vi "Transplantation_of_Description_field.vi"() -> ()   [LabVIEW 2018]
panel:
  out "error out":errorcluster
  in  "TDMS acceptor path":path
  in  "TDMS donor path":path
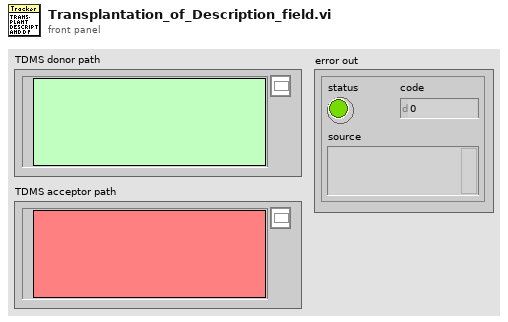
[diagram p1: front panel]
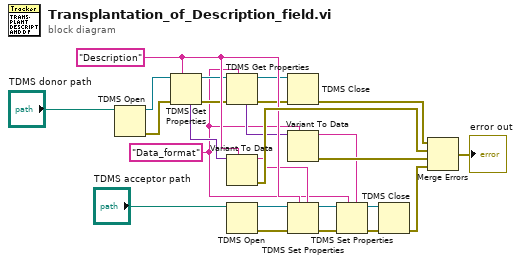
[diagram p0: block diagram]
diagram:
  w6 = "Data_format" ("property name")
  w16 = "Description" ("property name")
  n1 = TDMS Open(11:"TDMS donor path") -> (0:w24:errorcluster, 3:w25:refnum<k34>)  [unwired: 6 in]
  n2 = TDMS Get Properties(7:w16, 8:w24, 11:w25) -> (0:w11:errorcluster, 3:w13:refnum<k34>, 4:w22:variant)  [unwired: 3 in, 3 out]
  n3 = TDMS Get Properties(7:w6, 8:w11, 11:w13) -> (0:w10:errorcluster, 3:w12:refnum<k34>, 4:w9:variant)  [unwired: 3 in, 3 out]
  n4 = Variant To Data(type=w16, Variant=w22) -> (data=w15:string, error out=w20:errorcluster)  [unwired: 1 in]
  n5 = TDMS Open(11:"TDMS acceptor path") -> (0:w17:errorcluster, 3:w18:refnum<k34>)  [unwired: 6 in]
  n6 = TDMS Close(8:w10, 11:w12) -> (0:w23:errorcluster)  [unwired: 1 out]
  n7 = Variant To Data(type=w6, Variant=w9) -> (data=w5:string, error out=w7:errorcluster)  [unwired: 1 in]
  n8 = TDMS Set Properties(5:w15, 7:w16, 8:w17, 11:w18) -> (0:w3:errorcluster, 3:w4:refnum<k34>)  [unwired: 2 in, 2 out]
  n9 = TDMS Set Properties(5:w5, 7:w6, 8:w3, 11:w4) -> (0:w1:errorcluster, 3:w2:refnum<k34>)  [unwired: 2 in, 2 out]
  n10 = TDMS Close(8:w1, 11:w2) -> (0:w8:errorcluster)  [unwired: 1 out]
  n11 = Merge Errors(w23, w20, w7, w8) -> (→"error out":errorcluster)
